vi "KeepStreamLogicClassInMemory.vi"() -> (8 "Stream:StreamData.lvclass":refnum<class "StreamData.lvclass">, 10 "PipeLogic.lvclass":refnum<class "PipeLogic.lvclass">, 15 "Pipe.lvlib:PipeData.lvclass":refnum<class "StreamData.lvclass">)   [LabVIEW 2017, in "Stream-t'WPI_EncoderType.ctl'.lvlib"]
uses:
  <extravilib>/ChannelInstances/Stream-t'WPI_EncoderType.ctl'.lvlib
  <resource>/ChannelSupport/_ChannelSupport/PipeLogic/PipeLogic.lvclass
  <extravilib>/ChannelInstances/Stream-t'WPI_EncoderType.ctl'/StreamData.lvclass
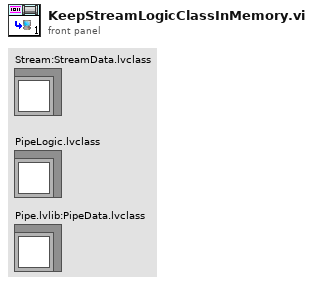
[diagram p1: front panel]
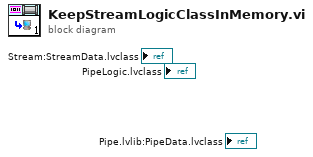
[diagram p0: block diagram]
diagram:
